vi "ESP32 Continuous Serial Write and Read.vi"() -> ()   [LabVIEW 2026]
doc: "This example performs writes and reads on a serial port, as directed by the user. You can press the Write and Read buttons, and change the Read Count, while the example is running.\n\nThe parameters set for the serial port must match the parameters of the connected instrument or device. In this example, the Read Count parameter specifies the number of bytes that the serial port reads. If there were more bytes at the port than the specified number, those bytes would not be read. If there were less bytes at the port than the specified number, you would receive a timeout error.\n\nThis example expands upon the flow control options for XON and XOFF, allowing the user to choose those control characters. Also, the user can enable or disable a termination character. Some devices require a termination character in order to identify the end of command strings. Some devices send a termination character to signify the end of data to be read. This example shows how you can end the Read operation once a termination character is detected in the buffer and/or append a termination character at the end of the Write data."
uses:
  Serial - Settings.ctl
  Control 1.ctl
  ESP32-PSOC-State Machine-1.ctl
  <vilib>/Instr/_visa.llb/VISA Flush IO Buffer Mask.ctl
  <vilib>/Instr/_visa.llb/VISA Configure Serial Port (Instr).vi
panel:
  in  "Command R":bool
  out "error":bool
  out "Connected":bool
  out "Serial Settings:Number of Bytes at Serial Port":u32
  out "Response 2":string
  in  "Command B":bool
  in  "Command A":bool
  in  "Toggle LED":bool
  in  "Enum":T1
  in  "Termination Character":u8=10 format="%.0x"
  in  "End Write on Termination Character?":bool=TRUE
  in  "Stop":bool
  out "Read Count":u32=1000
  out "Response":string
  in  "XON/XOFF Characters":T2={"XON"=enum."DC1", "XOFF"=enum."DC3"}
  in  "Serial Settings":T3={"baud rate"=115200, "data bits"=8, "parity"=enum."None", "stop bits"=10, "flow control"=0} {"flow control" items=["None"=0, "XON/XOFF"=1, "RTS/CTS"=2, "DTR/DSR"=4]; "stop bits" items=["1.0"=10, "1.5"=15, "2.0"=20]; "data bits" min=5 max=8 step=1; "baud rate" items=["75"=75, "110"=110, "134"=134, "150"=150, "300"=300, "600"=600, "1200"=1200, "1800"=1800, "2400"=2400, "4800"=4800, "7200"=7200, "9600"=9600, "14400"=14400, "19200"=19200, "28800"=28800, "38400"=38400, "56000"=56000, "57600"=57600, "115200"=115200, "128000"=128000, "230400"=230400]}
  in  "End Read on Termination Character?":bool=TRUE
  in  "VISA resource name":refnum<visa-resource-name>="COM3"
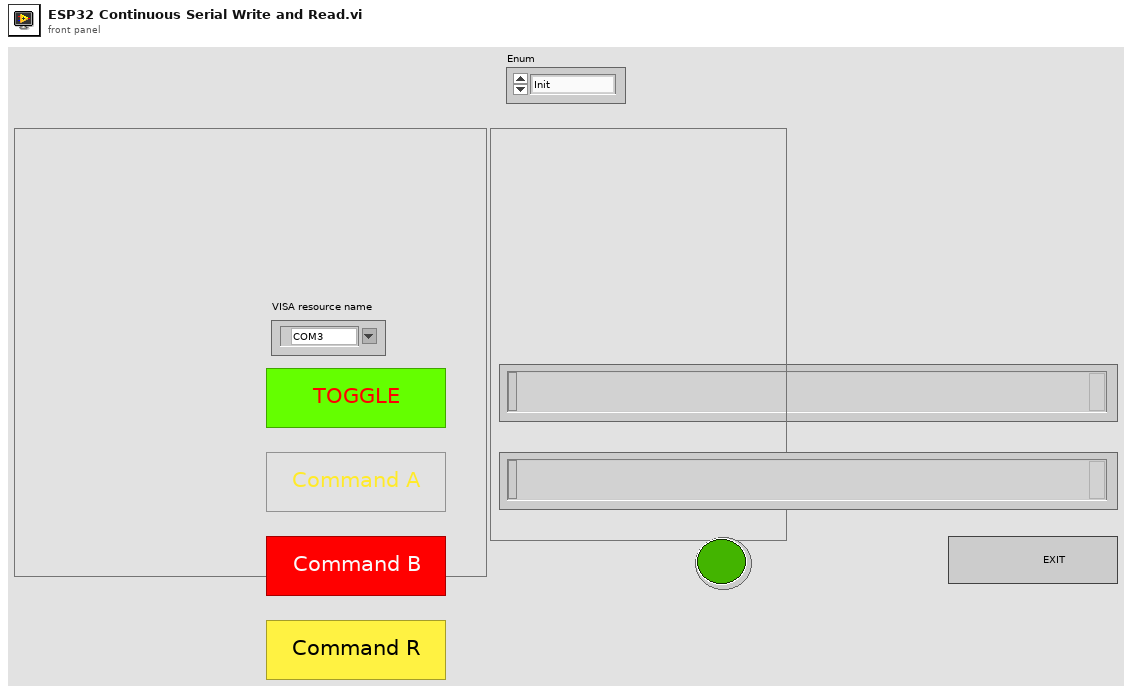
[diagram p1: front panel]
types:
  T1 = typedef "ESP32-PSOC-State Machine-1.ctl" = enum8{"Init", "Connect", "idle", "send", "wait", "receive", "que", "error", "exit"}
  T2 = typedef "Control 1.ctl" = cluster{"XON":enum16{"NUL", "SOH", "STX", "ETX", "EOT", "ENQ", "ACK", "BEL", "BS", "HT", "LF", "VT", "FF", "CR", "SO", "SI", "DLE", "DC1", "DC2", "DC3", "DC4", "NAK", "SYN", "ETB", "CAN", "EM", "SUB", "ESC", "FS", "GS", "RS", "US", "SP", "!", "\"", "#", "$", "%", "&", "'", "(", ")", "*", "+", ",", "- (-)", ".", "/", "0", "1", "2", "3", "4", "5", "6", "7", "8", "9", ":", ";", "<", "=", ">", "?", "@", "A", "B", "C", "D", "E", "F", "G", "H", "I", "J", "K", "L", "M", "N", "O", "P", "Q", "R", "S", "T", "U", "V", "W", "X", "Y", "Z", "[", "\\", "]", "^", "_", "`", "a", "b", "c", "d", "e", "f", "g", "h", "i", "j", "k", "l", "m", "n", "o", "p", "q", "r", "s", "t", "u", "v", "w", "x", "y", "z", "{", "|", "}", "~"}, "XOFF":enum16{"NUL", "SOH", "STX", "ETX", "EOT", "ENQ", "ACK", "BEL", "BS", "HT", "LF", "VT", "FF", "CR", "SO", "SI", "DLE", "DC1", "DC2", "DC3", "DC4", "NAK", "SYN", "ETB", "CAN", "EM", "SUB", "ESC", "FS", "GS", "RS", "US", "SP", "!", "\"", "#", "$", "%", "&", "'", "(", ")", "*", "+", ",", "- (-)", ".", "/", "0", "1", "2", "3", "4", "5", "6", "7", "8", "9", ":", ";", "<", "=", ">", "?", "@", "A", "B", "C", "D", "E", "F", "G", "H", "I", "J", "K", "L", "M", "N", "O", "P", "Q", "R", "S", "T", "U", "V", "W", "X", "Y", "Z", "[", "\\", "]", "^", "_", "`", "a", "b", "c", "d", "e", "f", "g", "h", "i", "j", "k", "l", "m", "n", "o", "p", "q", "r", "s", "t", "u", "v", "w", "x", "y", "z", "{", "|", "}", "~"}}
  T3 = typedef "Serial - Settings.ctl" = cluster{"baud rate":u32, "data bits":u16, "parity":enum16{"None", "Odd", "Even", "Mark", "Space"}, "stop bits":u16, "flow control":u16}
  T4 = enum16{"NUL", "SOH", "STX", "ETX", "EOT", "ENQ", "ACK", "BEL", "BS", "HT", "LF", "VT", "FF", "CR", "SO", "SI", "DLE", "DC1", "DC2", "DC3", "DC4", "NAK", "SYN", "ETB", "CAN", "EM", "SUB", "ESC", "FS", "GS", "RS", "US", "SP", "!", "\"", "#", "$", "%", "&", "'", "(", ")", "*", "+", ",", "- (-)", ".", "/", "0", "1", "2", "3", "4", "5", "6", "7", "8", "9", ":", ";", "<", "=", ">", "?", "@", "A", "B", "C", "D", "E", "F", "G", "H", "I", "J", "K", "L", "M", "N", "O", "P", "Q", "R", "S", "T", "U", "V", "W", "X", "Y", "Z", "[", "\\", "]", "^", "_", "`", "a", "b", "c", "d", "e", "f", "g", "h", "i", "j", "k", "l", "m", "n", "o", "p", "q", "r", "s", "t", "u", "v", "w", "x", "y", "z", "{", "|", "}", "~"}
  T5 = typedef "VISA Flush IO Buffer Mask.ctl" = u16
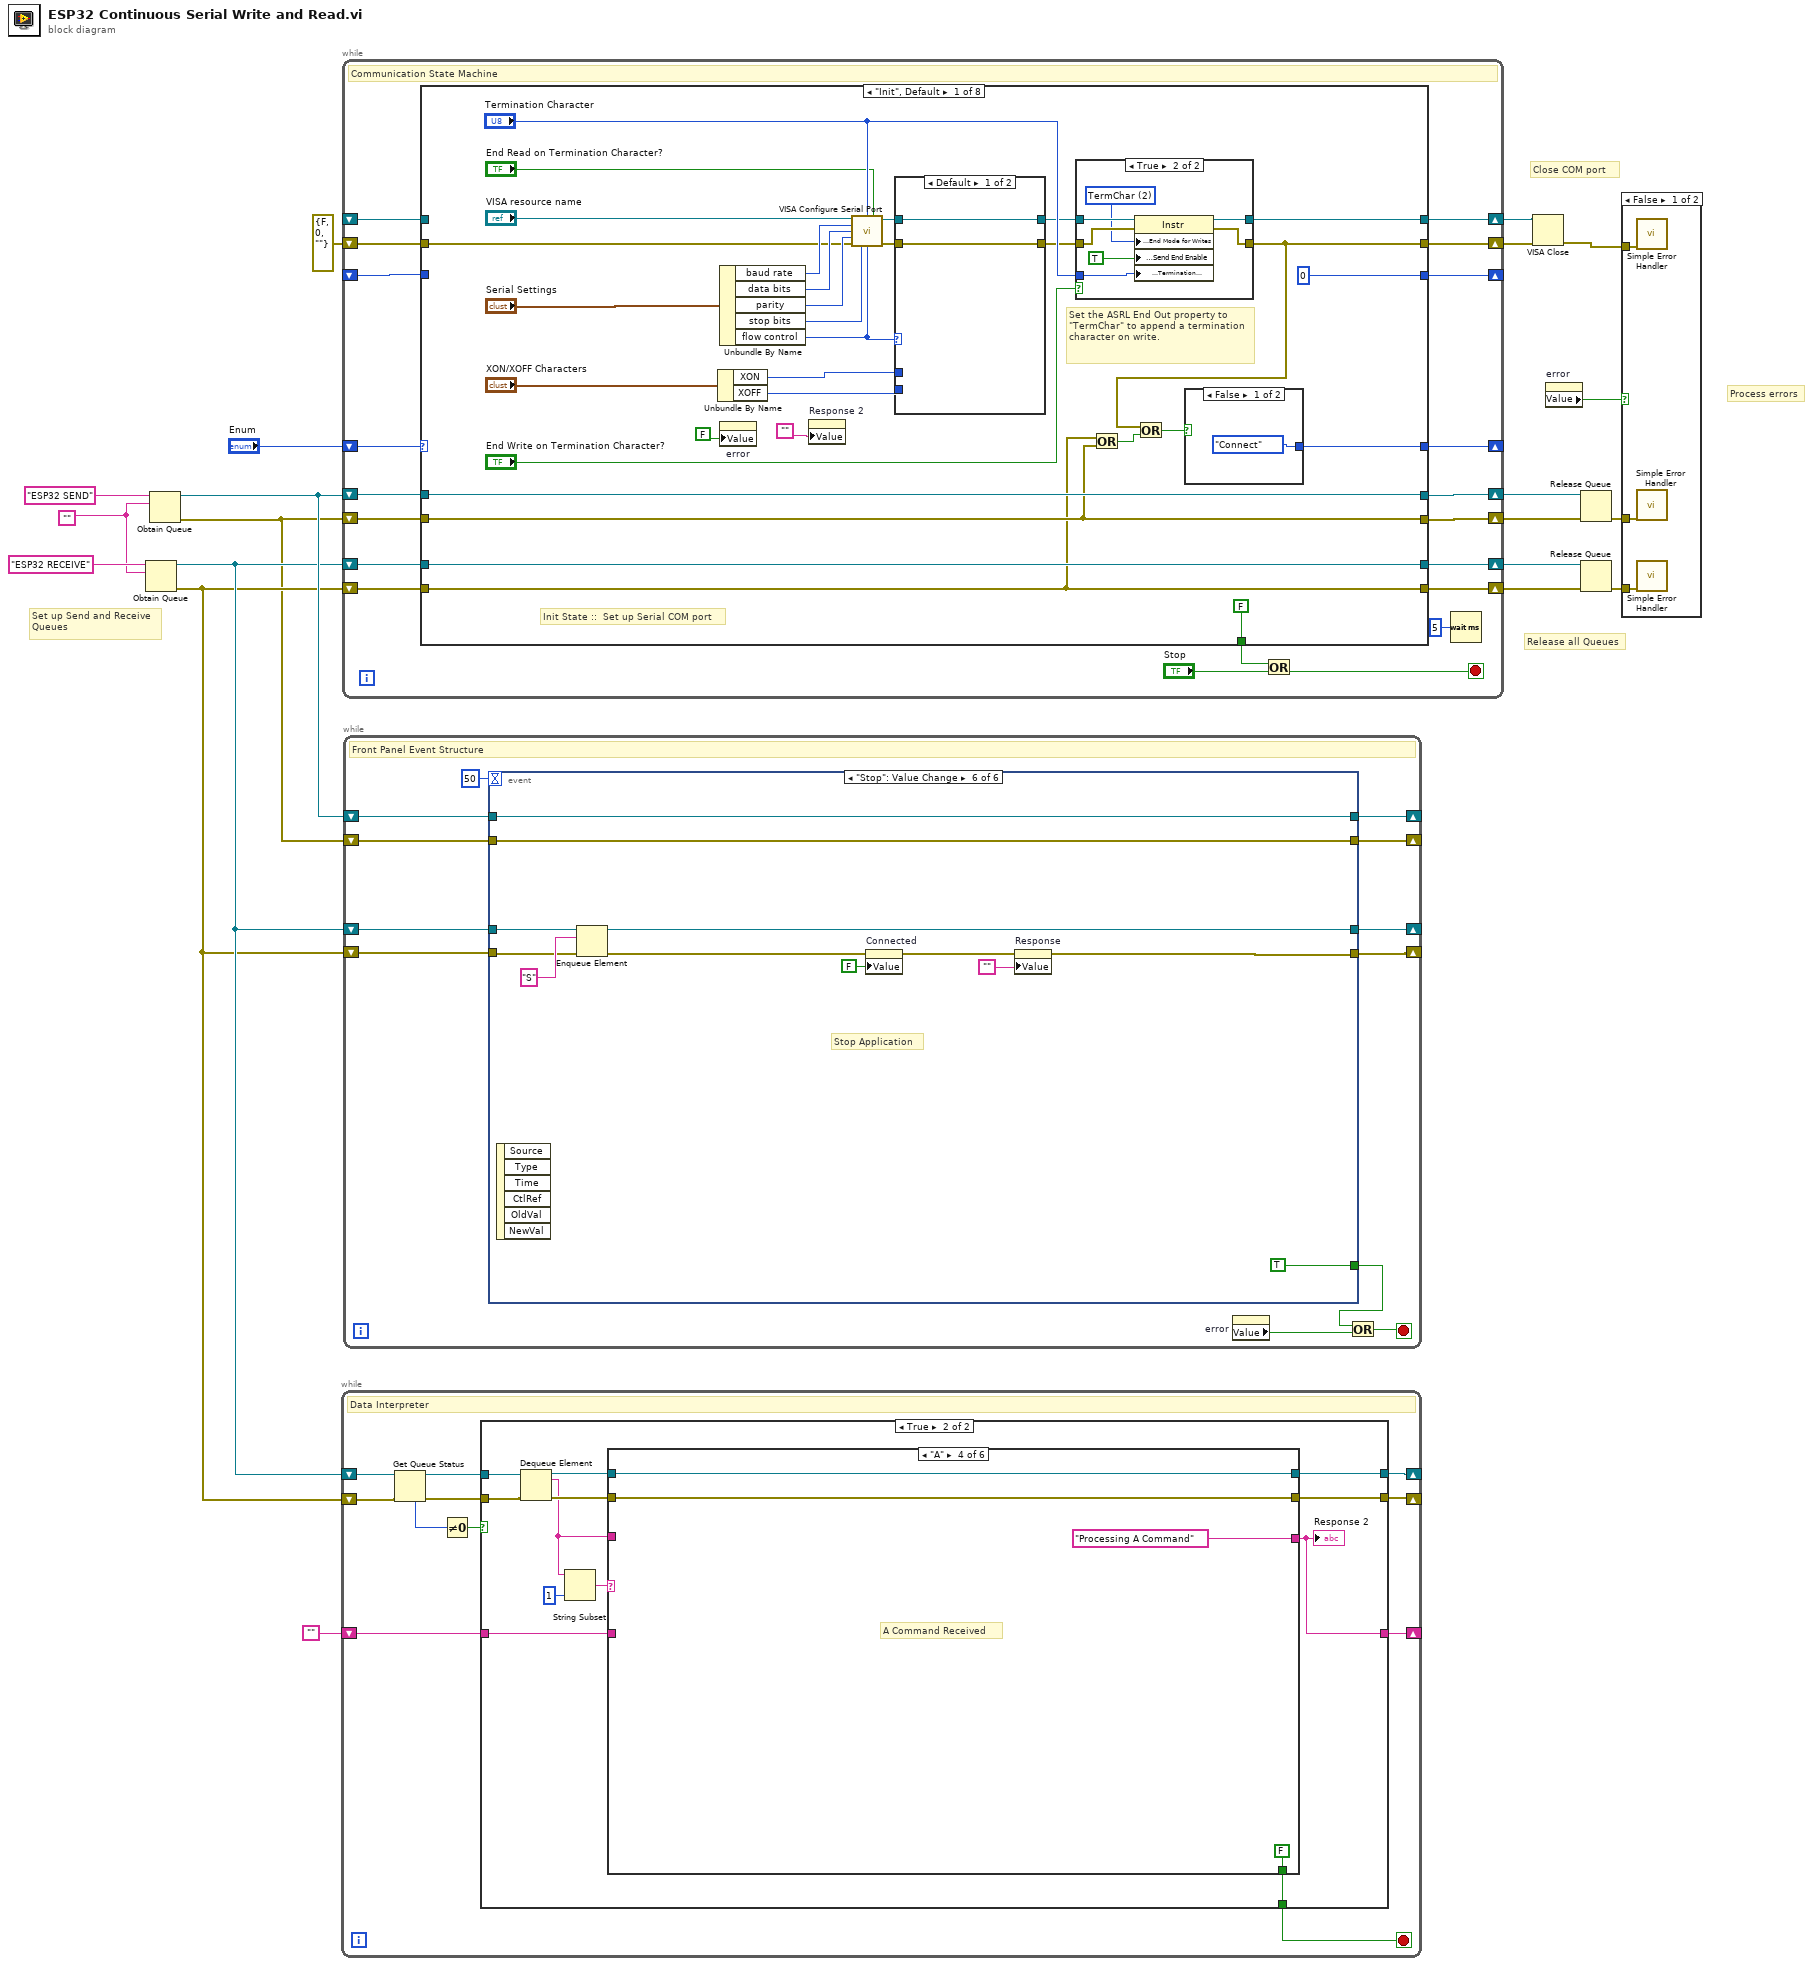
[diagram p0: block diagram]
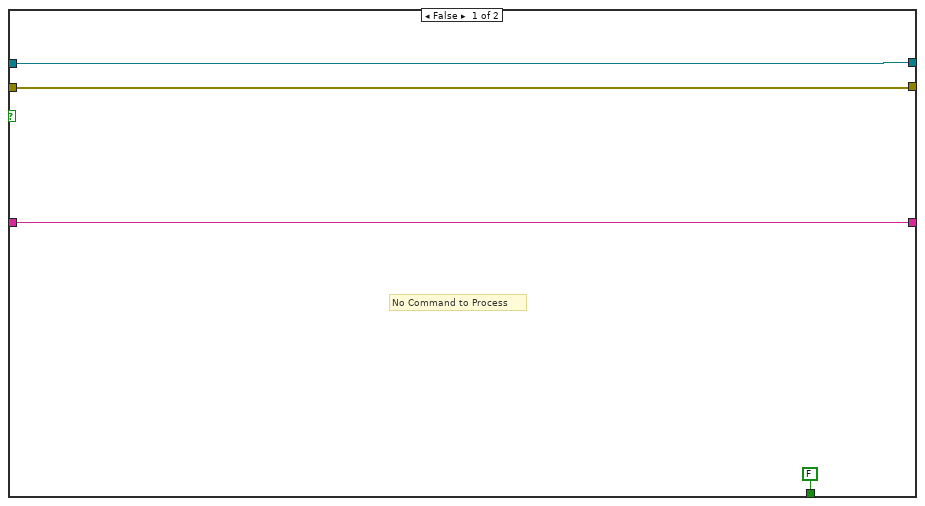
[diagram p3: hidden frame]
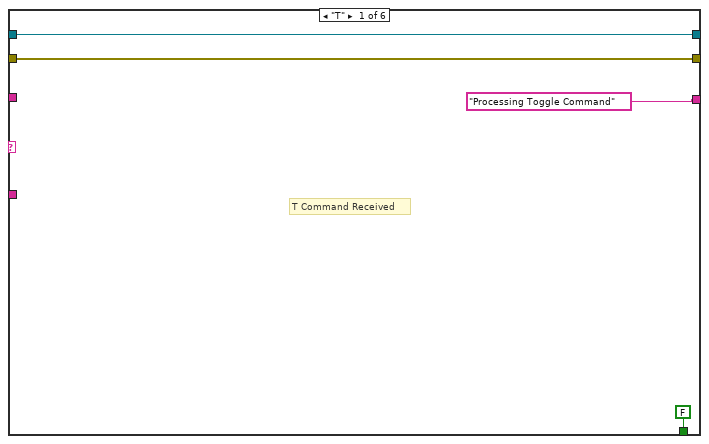
[diagram p4: hidden frame]
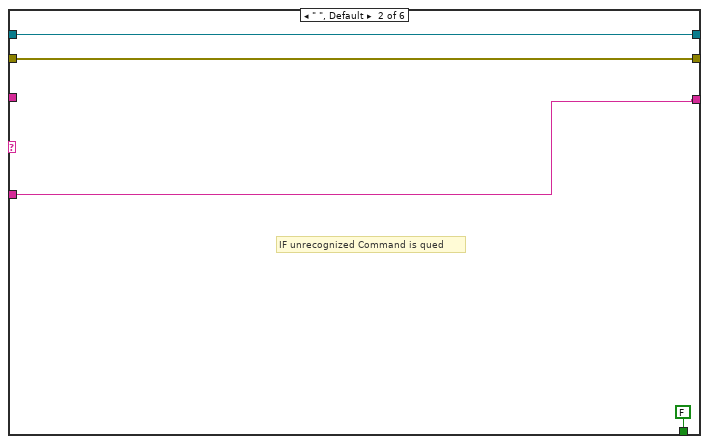
[diagram p5: hidden frame]
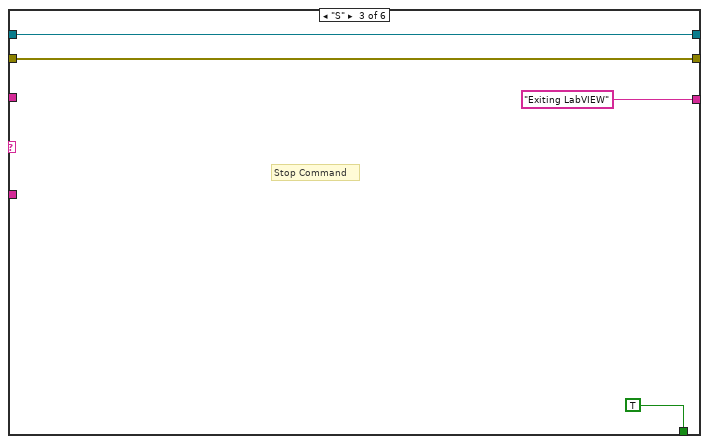
[diagram p6: hidden frame]
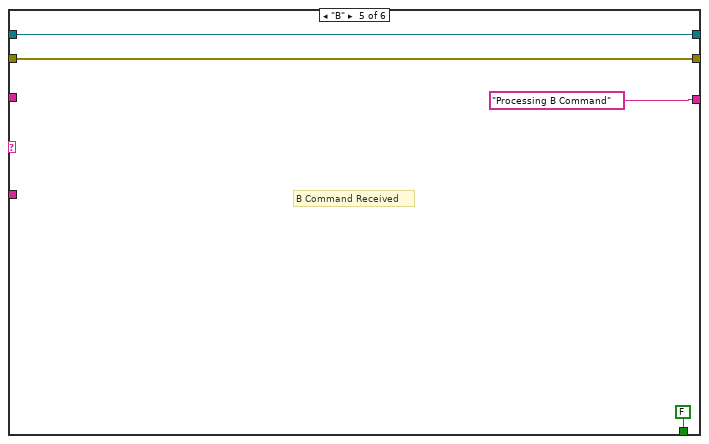
[diagram p7: hidden frame]
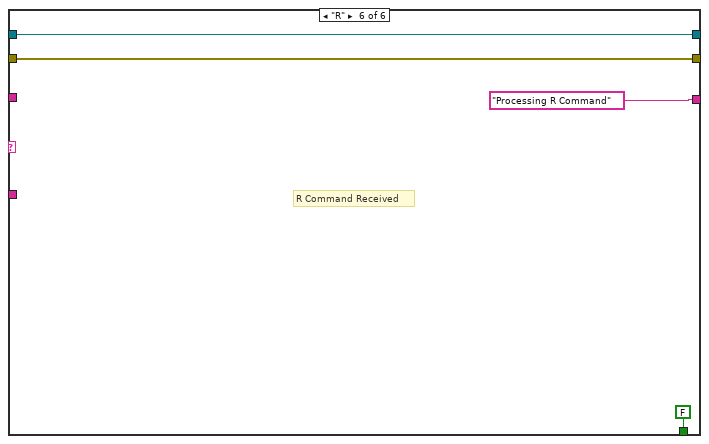
[diagram p8: hidden frame]
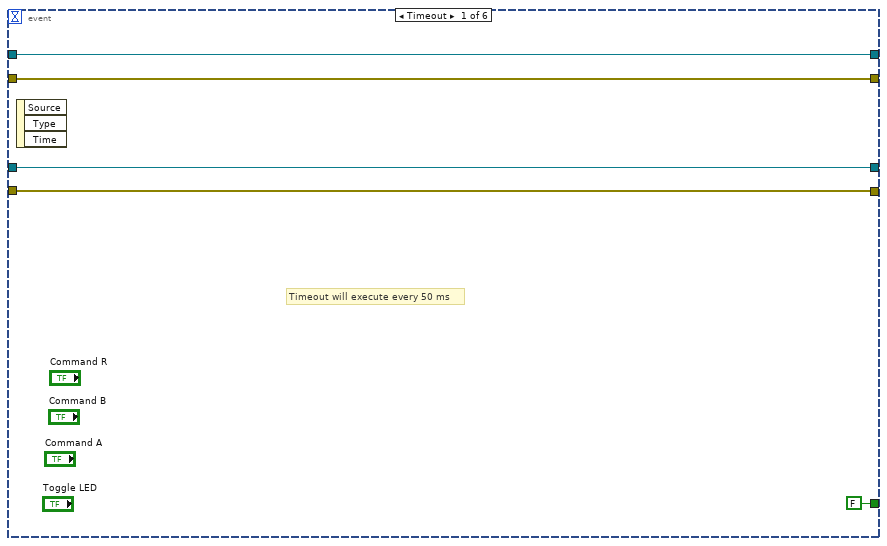
[diagram p9: hidden frame]
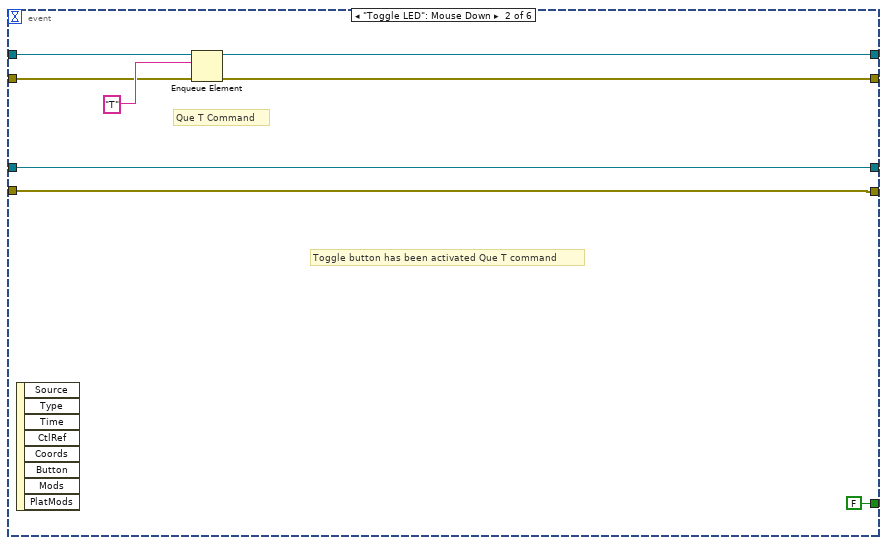
[diagram p10: hidden frame]
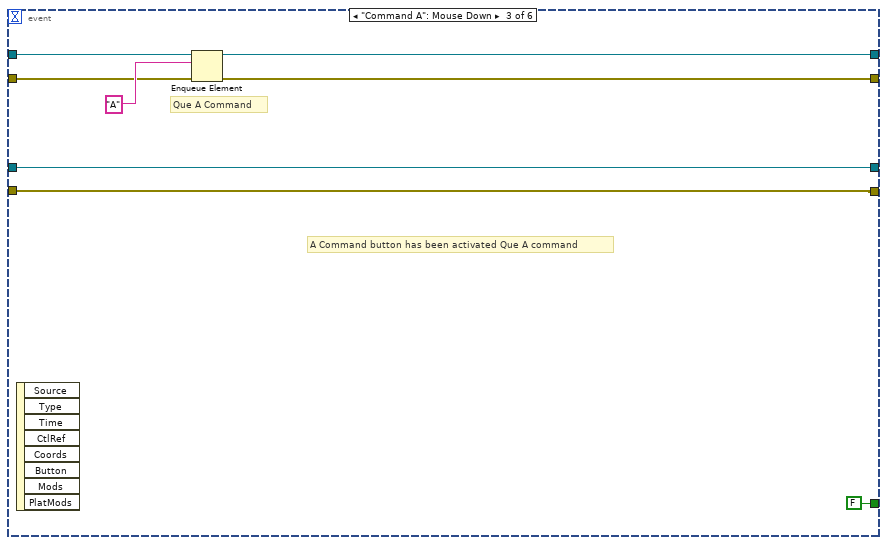
[diagram p11: hidden frame]
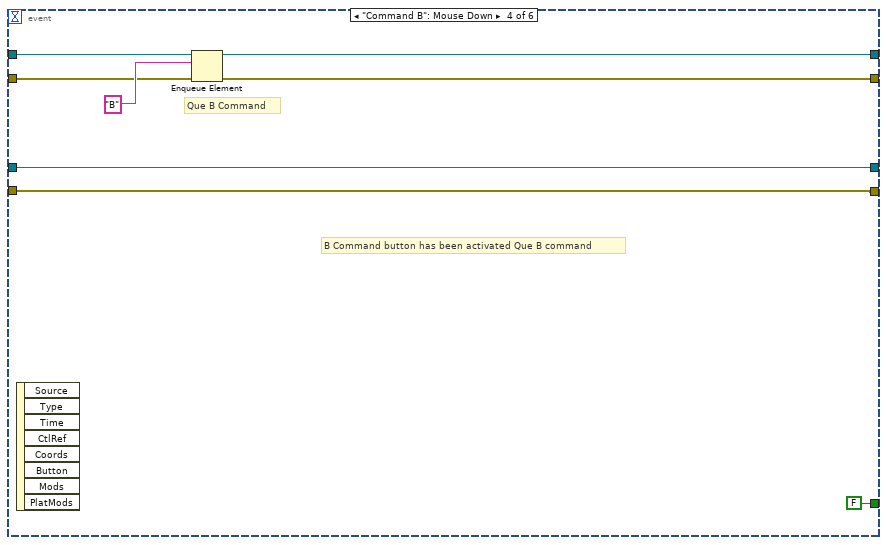
[diagram p12: hidden frame]
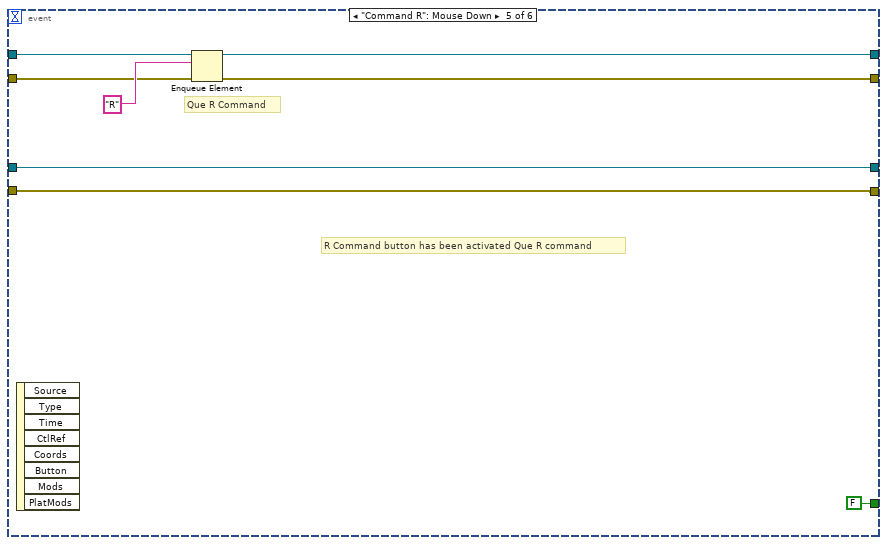
[diagram p13: hidden frame]
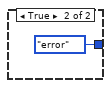
[diagram p14: hidden frame]
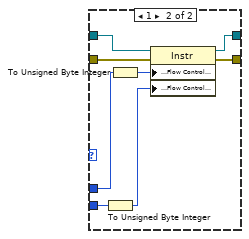
[diagram p16: hidden frame]
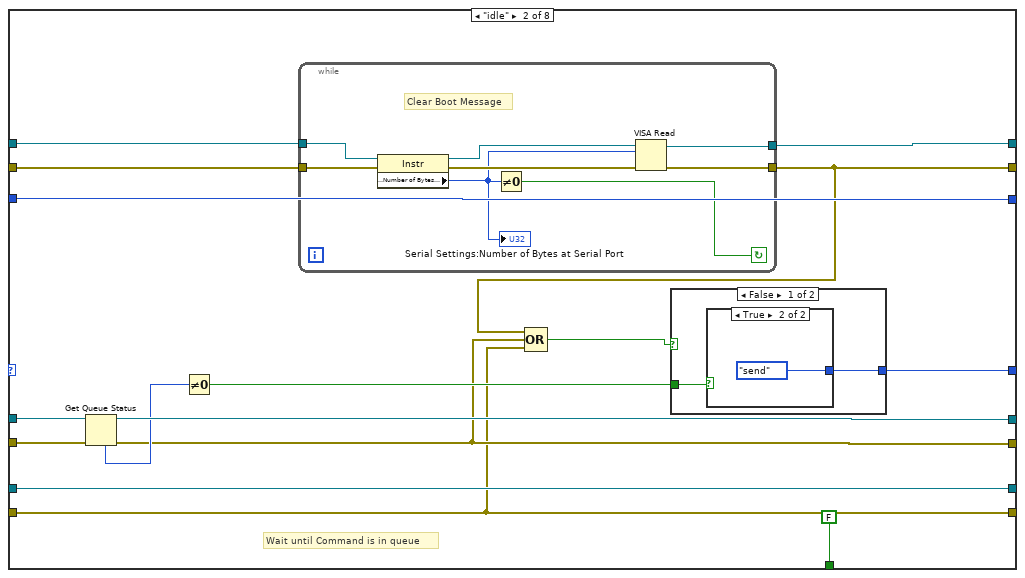
[diagram p17: hidden frame]
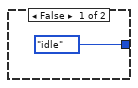
[diagram p18: hidden frame]
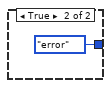
[diagram p19: hidden frame]
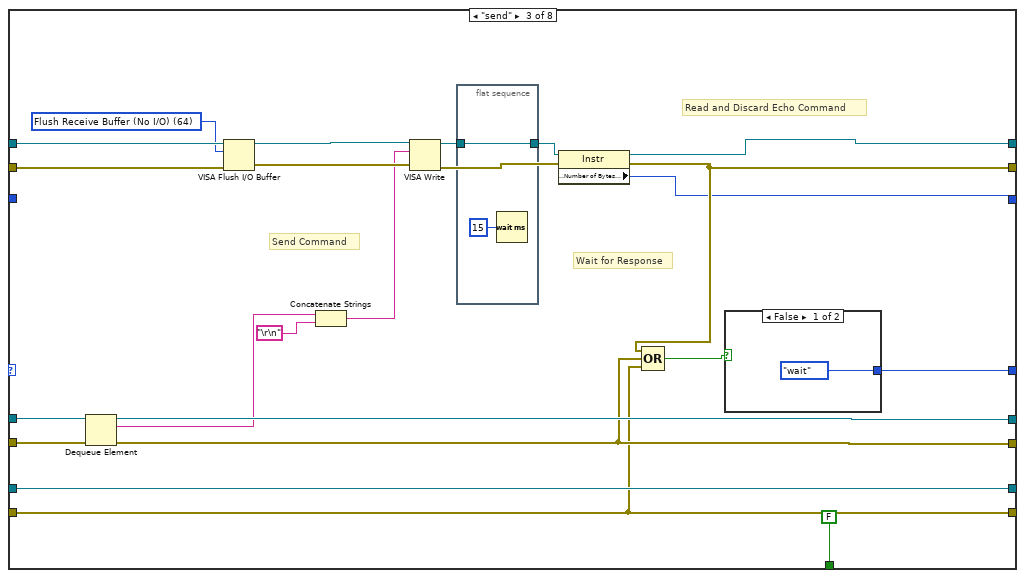
[diagram p20: hidden frame]
diagram:
  w10 = ""
  # "Process errors"
  # "Release all Queues"
  # "Close COM port"
  # "Set up Send and Receive\nQueues"
  n1 = Obtain Queue(name (unnamed)="ESP32 RECEIVE", element data type=w10) -> (queue out=w9:refnum<queue>, error out=w8:errorcluster)  [unwired: 3 in, 1 out]
  n2 = Obtain Queue(name (unnamed)="ESP32 SEND", element data type=w10) -> (queue out=w12:refnum<queue>, error out=w2:errorcluster)  [unwired: 3 in, 1 out]
  n3 = while {
    shift-right: [w25] -> _
    shift-left: w9 -> [w31]
    shift-right: [w24] -> _
    shift-left: w8 -> [w30]
    shift-right: [w22] -> _
    shift-left: "" -> [w21]
    stop <- w23 stop-if-true
    # "Data Interpreter"
    n4 = Get Queue Status(queue=w31, error in (no error)=w30) -> (queue out=w27:refnum<queue>, error out=w26:errorcluster, # elements in queue=w29:i32)  [unwired: 1 in, 5 out]
    n5 = Not Equal To 0?(x=w29) -> (x != 0?=w28:bool)
    n6 = case shown="True" w28 {
      tunnel: w27 -> [w35 w47]
      tunnel: w26 -> [w34 w46]
      tunnel: [w35 w41] -> w25
      tunnel: [w34 w40] -> w24
      tunnel: [FALSE w39] -> w23
      tunnel: [w32 w37] -> w22
      tunnel: w21 -> [w32 w36]
      frame False {
        # "No Command to Process"
      }
      frame True {
        n7 = Dequeue Element(queue=w47, error in (no error)=w46) -> (queue out=w45:refnum<queue>, element=w38:string, error out=w44:errorcluster)  [unwired: 1 in, 1 out]
        n8 = String Subset(string=w38, length (rest)=1 ("length (rest)")) -> (substring=w42:string)  [unwired: 1 in]
        n9 = case shown="\"A\"" w42 {
          tunnel: w45 -> [w51 w55 w59 w63 w67 w71]
          tunnel: w44 -> [w50 w54 w58 w62 w66 w70]
          tunnel: [w51 w55 w59 w63 w67 w71] -> w41
          tunnel: [w50 w54 w58 w62 w66 w70] -> w40
          tunnel: w38 -> [_ _ _ _ _ _]
          tunnel: [FALSE FALSE TRUE FALSE FALSE FALSE] -> w39
          tunnel: ["Processing Toggle Command" w52 "Exiting LabVIEW" "Processing A Command" "Processing B Command" "Processing R Command"] -> w37
          tunnel: w36 -> [_ w52 _ _ _ _]
          frame "T" {
            # "T Command Received"
          }
          frame " ", Default {
            # "IF unrecognized Command is qued"
          }
          frame "S" {
            # "Stop Command"
          }
          frame "A" {
            # "A Command Received"
          }
          frame "B" {
            # "B Command Received"
          }
          frame "R" {
            # "R Command Received"
          }
        }
        "Response 2" <- w37
      }
    }
  }
  n10 = while {
    shift-right: [w83] -> w20
    shift-left: w12 -> [w91]
    shift-right: [w82] -> w18
    shift-left: w2 -> [w90]
    shift-right: [w81] -> w19
    shift-left: w9 -> [w89]
    shift-right: [w80] -> w15
    shift-left: w8 -> [w88]
    shift-right: [w75] -> _
    shift-left: "Enum" -> [w74]
    shift-right: [w87] -> w14
    shift-left: _ -> [w84]
    shift-right: [w86] -> w13
    shift-left: errorcluster {"status"=FALSE, "code"=0, "source"=""} ("error out") -> [w85]
    shift-right: [w79] -> _
    shift-left: _ -> [w78]
    stop <- w73 stop-if-true
    # "Communication State Machine"
    n11 = case shown="\"Init\", Default" w74 {
      selector: w74 -> [_ _ _ _ _ _ w286 _]
      tunnel: [w121 w157 w193 w210 w248 w270 w285 w308] -> w83
      tunnel: [w95 w147 w185 w204 w231 w267 w284 w307] -> w82
      tunnel: [w101 w155 w186 w213 w249 ESP32-PSOC-State_Machine-1."exit" ("Enum") w286 ESP32-PSOC-State_Machine-1."idle" ("Enum")] -> w75
      tunnel: w91 -> [w121 w159 w195 w210 w248 w270 w285 w308]
      tunnel: w90 -> [w95 w158 w194 w204 w231 w267 w284 w307]
      tunnel: w89 -> [w122 w153 w192 w207 w243 w269 w283 w306]
      tunnel: w88 -> [w94 w146 w184 w203 w230 w266 w274 w305]
      tunnel: [w103 w150 w181 w212 w239 w272 w289 w310] -> w87
      tunnel: [w97 w148 w179 w205 w232 w268 w288 w311] -> w86
      tunnel: w85 -> [w99 w149 w189 w211 w234 w268 w288 w312]
      tunnel: w84 -> [_ w151 w191 w201 w246 w272 w289 w313]
      tunnel: [w122 w153 w192 w207 w241 w269 w281 w306] -> w81
      tunnel: [w94 w146 w184 w203 w242 w266 w277 w305] -> w80
      tunnel: [u32 0 ("Bytes at Port") w152 w173 w209 w244 w271 w287 w309] -> w79
      tunnel: w78 -> [_ w152 _ _ w222 w271 w287 w309]
      tunnel: [FALSE FALSE FALSE FALSE FALSE FALSE TRUE FALSE] -> w72
      frame "Init", Default {
        # "Init State ::  Set up Serial COM port"
        # "Set the ASRL End Out property to \"TermChar\" to append a termination character on write."
        n12 = Unbundle By Name("XON/XOFF Characters") -> ("XON"=w115:T4, "XOFF"=w116:T4)
        n13 = Unbundle By Name("Serial Settings") -> ("baud rate"=w111:u32, "data bits"=w110:u16, "parity"=w109:enum16{"None", "Odd", "Even", "Mark", "Space"}, "stop bits"=w108:u16, "flow control"=w114:u16)
        n14 = property on="error" class="Bool (strict)"("Value"=FALSE ("error")) -> ()  [unwired: 2 in, 2 out]
        n15 = property on="Response 2" class="Str"("Value"="") -> ()  [unwired: 2 in, 2 out]
        n16 = call-poly "VISA Configure Serial Port"("VISA resource name"="VISA resource name", "termination char\n(0xA = '\\n' = LF)"="Termination Character", "Enable Termination\nChar (T)"="End Read on Termination Character?", "baud rate (9600)"=w111, "data bits (8)"=w110, "parity (0:none)"=w109, "error in (no error)"=w99, "stop bits (10: 1 bit)"=w108, "flow control (0:none)"=w114) -> ("VISA resource name out"=w107:refnum<visa-resource-name>, "error out"=w106:errorcluster)  [unwired: 1 in, 4 out]
        n17 = case shown="Default" w114 {
          tunnel: [w134 w143] -> w117
          tunnel: [w135 w142] -> w118
          tunnel: w106 -> [w134 w141]
          tunnel: w107 -> [w135 w140]
          tunnel: w115 -> [_ w139]
          tunnel: w116 -> [_ w138]
          frame Default {
          }
          frame 1 {
            n18 = To Unsigned Byte Integer(number=w138) -> (unsigned 8bit integer=w137:u8)
            n19 = To Unsigned Byte Integer(number=w139) -> (unsigned 8bit integer=w136:u8)
            n20 = property class="Instr"(reference=w140, error in=w141, "Serial Settings:Flow Control XON Character"=w136, "Serial Settings:Flow Control XOFF Character"=w137) -> (reference out=w142:refnum<visa-resource-name>, error out=w143:errorcluster)
          }
        }
        n21 = case shown="True" "End Write on Termination Character?" {
          tunnel: w118 -> [w125 w133]
          tunnel: w117 -> [w126 w132]
          tunnel: [w125 w131] -> w103
          tunnel: [w126 w130] -> w97
          tunnel: "Termination Character" -> [_ w128]
          frame False {
          }
          frame True {
            w129 = u16 2 items=["None", "LastBit", "TermChar", "Break"] ("Serial Settings:Serial End Mode for Writes")
            n22 = property class="Instr"(reference=w133, error in=w132, "Serial Settings:End Mode for Writes"=w129, "Message Based Settings:Send End Enable"=TRUE, "Message Based Settings:Termination Character"=w128) -> (reference out=w131:refnum<visa-resource-name>, error out=w130:errorcluster)
          }
        }
        n23 = Or(x=w94, y=w95) -> (x .or. y?=w96:bool)
        n24 = Or(x=w97, y=w96) -> (x .or. y?=w98:bool)
        n25 = case shown="False" w98 {
          tunnel: [ESP32-PSOC-State_Machine-1."Connect" ("Enum") ESP32-PSOC-State_Machine-1."error" ("Enum")] -> w101
          frame False {
          }
          frame True {
          }
        }
      }
      frame "idle" {
        # "Wait until Command is in queue"
        n26 = Get Queue Status(queue=w159, error in (no error)=w158) -> (queue out=w157:refnum<queue>, error out=w147:errorcluster, # elements in queue=w156:i32)  [unwired: 1 in, 5 out]
        n27 = Not Equal To 0?(x=w156) -> (x != 0?=w154:bool)
        n28 = while {
          tunnel: w151 -> [w172]
          tunnel: [w168] -> w150
          tunnel: w149 -> [w171]
          tunnel: [w166] -> w148
          stop <- w170 continue-if-true
          # "Clear Boot Message"
          n29 = property class="Instr"(reference=w172, error in=w171) -> (reference out=w169:refnum<visa-resource-name>, error out=w167:errorcluster, "Serial Settings:Number of Bytes at Serial Port"=w165:u32)
          "Serial Settings:Number of Bytes at Serial Port" <- w165
          n30 = Not Equal To 0?(x=w165) -> (x != 0?=w170:bool)
          n31 = VISA Read(VISA resource name=w169, byte count=w165, error in (no error)=w167) -> (VISA resource name out=w168:refnum<visa-resource-name>, error out=w166:errorcluster)  [unwired: 2 out]
        }
        n32 = Compound Arithmetic op=OR(w148, w147, w146) -> (w145:bool)
        n33 = case shown="False" w145 {
          tunnel: [w161 ESP32-PSOC-State_Machine-1."error" ("Enum")] -> w155
          tunnel: w154 -> [w160 _]
          frame False {
            n34 = case shown="True" w160 {
              tunnel: [ESP32-PSOC-State_Machine-1."idle" ("Enum") ESP32-PSOC-State_Machine-1."send" ("Enum")] -> w161
              frame False {
              }
              frame True {
              }
            }
          }
          frame True {
          }
        }
      }
      frame "send" {
        w187 = T5 64 items=["Flush Receive Buffer"=16, "Write Transmit Buffer to Device"=32, "Flush Receive Buffer (No I/O)"=64, "Flush Transmit Buffer"=128] ("Mask")
        # "Read and Discard Echo Command"
        # "Wait for Response"
        # "Send Command"
        n35 = Dequeue Element(queue=w195, error in (no error)=w194) -> (queue out=w193:refnum<queue>, element=w177:string, error out=w185:errorcluster)  [unwired: 1 in, 1 out]
        n36 = VISA Flush I/O Buffer(VISA resource name=w191, mask (16)=w187, error in (no error)=w189) -> (VISA resource name out=w190:refnum<visa-resource-name>, error out=w188:errorcluster)
        n37 = Concatenate Strings(w177, "\r\n") -> (w176:string)
        n38 = VISA Write(VISA resource name=w190, write buffer=w176, error in (no error)=w188) -> (VISA resource name out=w175:refnum<visa-resource-name>, error out=w180:errorcluster)  [unwired: 1 out]
        n39 = flat-sequence {
          tunnel: w175 -> [w197]
          tunnel: [w197] -> w174
          frame #0 {
            n40 = Wait (ms)(milliseconds to wait=u32 15) -> ()  [unwired: 1 out]
          }
        }
        n41 = property class="Instr"(reference=w174, error in=w180) -> (reference out=w181:refnum<visa-resource-name>, error out=w179:errorcluster, "Serial Settings:Number of Bytes at Serial Port"=w173:u32)
        n42 = Compound Arithmetic op=OR(w179, w185, w184) -> (w183:bool)
        n43 = case shown="False" w183 {
          tunnel: [ESP32-PSOC-State_Machine-1."wait" ("Enum") ESP32-PSOC-State_Machine-1."error" ("Enum")] -> w186
          frame False {
          }
          frame True {
          }
        }
      }
      frame "wait" {
        # "Wait for actual Response"
        n44 = flat-sequence {
          tunnel: w201 -> [w215]
          tunnel: [w215] -> w200
          frame #0 {
            n45 = Wait (ms)(milliseconds to wait=u32 15) -> ()  [unwired: 1 out]
          }
        }
        n46 = property class="Instr"(reference=w200, error in=w211) -> (reference out=w212:refnum<visa-resource-name>, error out=w205:errorcluster, "Serial Settings:Number of Bytes at Serial Port"=w209:u32)
        n47 = Not Equal To 0?(x=w209) -> (x != 0?=w208:bool)
        n48 = Compound Arithmetic op=OR(w205, w204, w203) -> (w206:bool)
        n49 = case shown="False" w206 {
          tunnel: [w217 ESP32-PSOC-State_Machine-1."error" ("Enum")] -> w213
          tunnel: w208 -> [w216 _]
          frame False {
            n50 = case shown="True" w216 {
              tunnel: [ESP32-PSOC-State_Machine-1."wait" ("Enum") ESP32-PSOC-State_Machine-1."receive" ("Enum")] -> w217
              frame False {
              }
              frame True {
              }
            }
          }
          frame True {
          }
        }
      }
      frame "receive" {
        # "Process Response and Display"
        # "Read Response"
        n51 = VISA Read(VISA resource name=w246, byte count=w222, error in (no error)=w234) -> (VISA resource name out=w240:refnum<visa-resource-name>, read buffer=w236:string, return count=w221:u32, error out=w245:errorcluster)
        n52 = String To Byte Array(string=w236) -> (unsigned byte array=w235:u8[])
        n53 = property class="Instr"(reference=w240, error in=w245) -> (reference out=w239:refnum<visa-resource-name>, error out=w233:errorcluster, "Serial Settings:Number of Bytes at Serial Port"=w244:u32)
        n54 = Index Array(array=w235, index=0) -> (element=w227:u8)
        n55 = Equal?(x=w227, y=u8 13) -> (x = y?=w225:bool)
        n56 = Equal?(x=w227, y=u8 10) -> (x = y?=w224:bool)
        n57 = Not Or(1:w224, 2:w225) -> (0:w223:bool)
        n58 = Not Equal To 0?(x=w244) -> (x != 0?=w247:bool)
        n59 = case shown="True" w223 {
          tunnel: w235 -> [_ w256]
          tunnel: w233 -> [w255 w258]
          tunnel: [w255 w257] -> w232
          tunnel: w221 -> [_ _]
          frame False {
          }
          frame True {
            (unwired) 1 ("length")
            (unwired) 0 ("index")
            n60 = property on="Response" class="Str"(error in=w258, "Value"="") -> (error out=w260:errorcluster)  [unwired: 1 in, 1 out]
            n61 = Byte Array To String(unsigned byte array=w256) -> (string=w259:string)
            n62 = property on="Response" class="Str"(error in=w260, "Value"=w259) -> (error out=w257:errorcluster)  [unwired: 1 in, 1 out]
          }
        }
        n63 = Compound Arithmetic op=OR(w232, w231, w230) -> (w229:bool)
        n64 = Enqueue Element(queue=w243, element=w236, error in (no error)=w230) -> (queue out=w241:refnum<queue>, error out=w242:errorcluster)  [unwired: 1 in, 1 out]
        n65 = case shown="False" w229 {
          tunnel: [w251 ESP32-PSOC-State_Machine-1."error" ("Enum")] -> w249
          tunnel: w247 -> [w250 _]
          frame False {
            n66 = case shown="True" w250 {
              tunnel: [ESP32-PSOC-State_Machine-1."idle" ("Enum") ESP32-PSOC-State_Machine-1."receive" ("Enum")] -> w251
              frame False {
              }
              frame True {
              }
            }
          }
          frame True {
          }
        }
        "Read Count" <- w222
      }
      frame "error" {
        # "Process any error"
        n67 = Build Array(w268, w267, w266) -> (w265:errorcluster[])
        n68 = for {
          tunnel: w265 -> [w273] mode=indexing
          n69 = call <vilib>:"General Error Handler.vi"("error in (no error)"=w273) -> ()  [unwired: 10 in, 5 out]
        }
        "error" <- TRUE ("error")
      }
      frame "exit" {
        # "Exit due to error"
        n70 = Enqueue Element(queue=w283, element="S", error in (no error)=w274) -> (queue out=w281:refnum<queue>, error out=w279:errorcluster)  [unwired: 1 in, 1 out]
        n71 = property on="Connected" class="Bool (strict)"(error in=w279, "Value"=FALSE ("Connected")) -> (error out=w278:errorcluster)  [unwired: 1 in, 1 out]
        n72 = property on="Response" class="Str"(error in=w278, "Value"="") -> (error out=w277:errorcluster)  [unwired: 1 in, 1 out]
      }
      frame "Connect" {
        # "Validating connection"
        # "Send ID to validate connection"
        # "Clear any residual characters"
        n73 = while {
          shift-right: [w337] -> w301
          shift-left: w312 -> [w343]
          shift-right: [w336] -> w302
          shift-left: w313 -> [w342]
          stop <- w341 continue-if-true
          n74 = property class="Instr"(reference=w342, error in=w343) -> (reference out=w339:refnum<visa-resource-name>, error out=w338:errorcluster, "Bytes at Port"=w335:u32)
          n75 = VISA Read(VISA resource name=w339, byte count=w335, error in (no error)=w338) -> (VISA resource name out=w336:refnum<visa-resource-name>, read buffer=w334:string, error out=w337:errorcluster)  [unwired: 1 out]
          n76 = Wait (ms)(milliseconds to wait=u32 5) -> ()  [unwired: 1 out]
          n77 = Search/Split String(string=w334, search string/char (-)="Commands") -> (match + rest of string=w332:string)  [unwired: 1 in, 2 out]
          n78 = String Length(string=w332) -> (length=w331:i32)
          n79 = Equal To 0?(x=w331) -> (x = 0?=w341:bool)
        }
        n80 = Concatenate Strings("I" ("write buffer"), "\r\n") -> (w290:string)
        n81 = VISA Write(VISA resource name=w302, write buffer=w290, error in (no error)=w301) -> (VISA resource name out=w296:refnum<visa-resource-name>, error out=w300:errorcluster)  [unwired: 1 out]
        n82 = flat-sequence {
          tunnel: w296 -> [w330]
          tunnel: [w330] -> w295
          frame #0 {
            n83 = Wait (ms)(milliseconds to wait=u32 5) -> ()  [unwired: 1 out]
          }
        }
        n84 = property class="Instr"(reference=w295, error in=w300) -> (reference out=w298:refnum<visa-resource-name>, error out=w299:errorcluster, "Bytes at Port"=w297:u32)
        n85 = VISA Read(VISA resource name=w298, byte count=w297, error in (no error)=w299) -> (VISA resource name out=w293:refnum<visa-resource-name>, error out=w294:errorcluster)  [unwired: 2 out]
        n86 = while {
          shift-right: [w317] -> w311
          shift-left: w294 -> [w323]
          shift-right: [w318] -> w310
          shift-left: w293 -> [w316]
          stop <- w314 stop-if-true
          n87 = flat-sequence {
            tunnel: w316 -> [w328]
            tunnel: [w328] -> w315
            frame #0 {
              n88 = Wait (ms)(milliseconds to wait=u32 15) -> ()  [unwired: 1 out]
            }
          }
          n89 = property class="Instr"(reference=w315, error in=w323) -> (reference out=w321:refnum<visa-resource-name>, error out=w322:errorcluster, "Bytes at Port"=w320:u32)
          n90 = VISA Read(VISA resource name=w321, byte count=w320, error in (no error)=w322) -> (VISA resource name out=w318:refnum<visa-resource-name>, read buffer=w319:string, error out=w317:errorcluster)  [unwired: 1 out]
          n91 = Search/Split String(string=w319, search string/char (-)="ESP32") -> (match + rest of string=w325:string)  [unwired: 1 in, 2 out]
          n92 = String Length(string=w325) -> (length=w324:i32)
          n93 = Not Equal To 0?(x=w324) -> (x != 0?=w314:bool)
          "Connected" <- w314
        }
      }
    }
    n94 = Or(x=w72, y="Stop") -> (x .or. y?=w73:bool)
    n95 = Wait (ms)(milliseconds to wait=u32 5) -> ()  [unwired: 1 out]
  }
  n96 = while {
    shift-right: [w352] -> _
    shift-left: w12 -> [w353]
    shift-right: [w351] -> _
    shift-left: w2 -> [w354]
    shift-right: [w347] -> _
    shift-left: w9 -> [w350]
    shift-right: [w348] -> _
    shift-left: w8 -> [w349]
    stop <- w344 stop-if-true
    # "Front Panel Event Structure"
    n97 = event shown="[5] \"Stop\": Value Change" {
      selector: _ -> [_ _ _ _ _ _]
      dyn-events: _ -> [_ _ _ _ _ _]
      timeout: 50 -> [_ _ _ _ _ _]
      tunnel: w354 -> [w359 w366 w374 w382 w390 w402]
      tunnel: w353 -> [w356 w368 w376 w384 w392 w403]
      tunnel: [w356 w365 w373 w381 w389 w403] -> w352
      tunnel: [w359 w364 w372 w380 w388 w402] -> w351
      tunnel: [FALSE FALSE FALSE FALSE FALSE TRUE] -> w346
      tunnel: w350 -> [w358 w362 w370 w378 w386 w401]
      tunnel: w349 -> [w357 w361 w369 w377 w385 w399]
      tunnel: [w357 w361 w369 w377 w385 w394] -> w348
      tunnel: [w358 w362 w370 w378 w386 w398] -> w347
      event Timeout {
        # "Timeout will execute every 50 ms"
        n98 = event-data() -> ()  [unwired: 1 in, 3 out]
      }
      event "Toggle LED": Mouse Down {
        # "Que T Command"
        # "Toggle button has been activated Que T command"
        n99 = event-data() -> ()  [unwired: 1 in, 8 out]
        n100 = Enqueue Element(queue=w368, element="T", error in (no error)=w366) -> (queue out=w365:refnum<queue>, error out=w364:errorcluster)  [unwired: 1 in, 1 out]
      }
      event "Command A": Mouse Down {
        # "Que A Command"
        # "A Command button has been activated Que A command"
        n101 = event-data() -> ()  [unwired: 1 in, 8 out]
        n102 = Enqueue Element(queue=w376, element="A", error in (no error)=w374) -> (queue out=w373:refnum<queue>, error out=w372:errorcluster)  [unwired: 1 in, 1 out]
      }
      event "Command B": Mouse Down {
        # "Que B Command"
        # "B Command button has been activated Que B command"
        n103 = event-data() -> ()  [unwired: 1 in, 8 out]
        n104 = Enqueue Element(queue=w384, element="B", error in (no error)=w382) -> (queue out=w381:refnum<queue>, error out=w380:errorcluster)  [unwired: 1 in, 1 out]
      }
      event "Command R": Mouse Down {
        # "Que R Command"
        # "R Command button has been activated Que R command"
        n105 = event-data() -> ()  [unwired: 1 in, 8 out]
        n106 = Enqueue Element(queue=w392, element="R", error in (no error)=w390) -> (queue out=w389:refnum<queue>, error out=w388:errorcluster)  [unwired: 1 in, 1 out]
      }
      event "Stop": Value Change {
        # "Stop Application"
        n107 = event-data() -> ()  [unwired: 1 in, 6 out]
        n108 = Enqueue Element(queue=w401, element="S", error in (no error)=w399) -> (queue out=w398:refnum<queue>, error out=w397:errorcluster)  [unwired: 1 in, 1 out]
        n109 = property on="Connected" class="Bool (strict)"(error in=w397, "Value"=FALSE ("Connected")) -> (error out=w395:errorcluster)  [unwired: 1 in, 1 out]
        n110 = property on="Response" class="Str"(error in=w395, "Value"="") -> (error out=w394:errorcluster)  [unwired: 1 in, 1 out]
      }
    }
    n111 = property on="error" class="Bool (strict)"() -> ("Value"=w345:bool)  [unwired: 2 in, 2 out]
    n112 = Or(x=w346, y=w345) -> (x .or. y?=w344:bool)
  }
  n113 = VISA Close(VISA resource name=w14, error in (no error)=w13) -> (error out=w5:errorcluster)
  n114 = property on="error" class="Bool (strict)"() -> ("Value"=w1:bool)  [unwired: 2 in, 2 out]
  n115 = Release Queue(queue=w20, error in (no error)=w18) -> (error out=w4:errorcluster)  [unwired: 1 in, 2 out]
  n116 = Release Queue(queue=w19, error in (no error)=w15) -> (error out=w3:errorcluster)  [unwired: 1 in, 2 out]
  n117 = case shown="False" w1 {
    tunnel: w5 -> [w407 _]
    tunnel: w4 -> [w406 _]
    tunnel: w3 -> [w405 _]
    frame False {
      n118 = call <vilib>:"Simple Error Handler.vi"("error in (no error)"=w407) -> ()  [unwired: 1 in, 8 out]
      n119 = call <vilib>:"Simple Error Handler.vi"("error in (no error)"=w406) -> ()  [unwired: 1 in, 8 out]
      n120 = call <vilib>:"Simple Error Handler.vi"("error in (no error)"=w405) -> ()  [unwired: 1 in, 8 out]
    }
    frame True {
    }
  }
